vi "Set Index.vi"(8 "error in (no error)":errorcluster, 10 "Index":i32, 11 "Array in":refnum<class "Vector Parent.lvclass">) -> (0 "error out":errorcluster, 3 "Array out":refnum<class "Vector Parent.lvclass">)   [LabVIEW 2021, in "Vector Parent.lvclass"]
uses:
  Vector Parent.lvclass
  Vector Parent.lvclass/Vector Parent.ctl
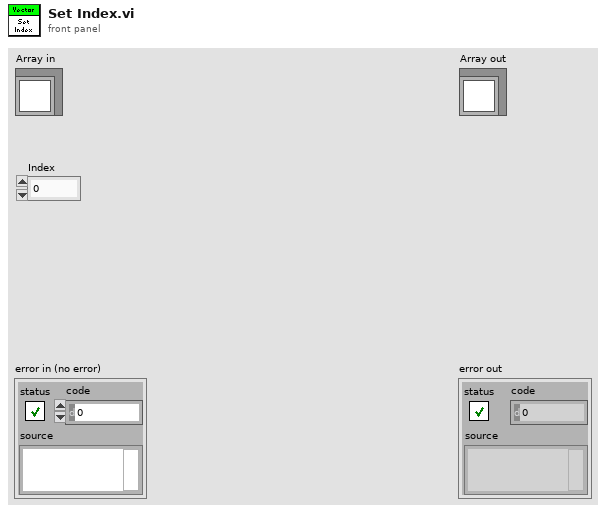
[diagram p1: front panel]
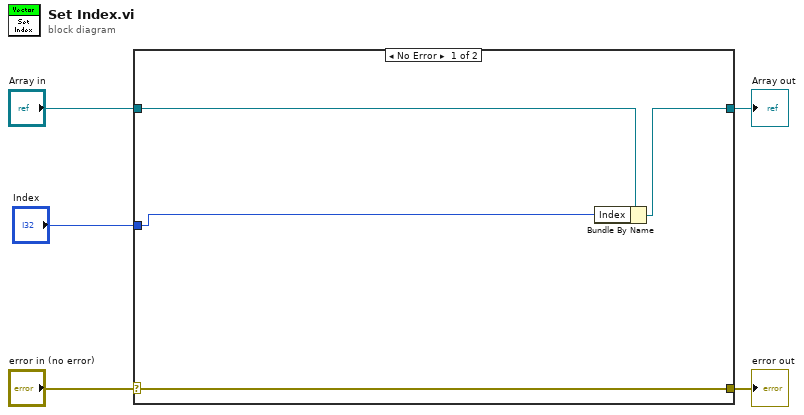
[diagram p0: block diagram]
diagram:
  n1 = case shown="No Error" "error in (no error)" {
    selector: "error in (no error)" -> [w9 w11]
    tunnel: [w9 w11] -> w4
    tunnel: [w7 w10] -> w2
    tunnel: "Array in" -> [w8 w10]
    tunnel: "Index" -> [w6 _]
    frame No Error {
      n2 = Bundle By Name(cluster=w8, "Index"=w6) -> (w7:refnum<class "Vector Parent.lvclass">)
    }
    frame Error {
    }
  }
  "error out" <- w4
  "Array out" <- w2
